vi "Create Status Queue.vi"(8 "error in (no error)":errorcluster, 11 "Test Step Controller.lvlib:Test Step Controller.lvclass":refnum<class "Server Controller.lvclass">) -> (0 "error out":errorcluster, 2 "queue out":refnum<queue>, 3 "Controller out":refnum<class "Server Controller.lvclass">)   [LabVIEW 2026, in "Server Controller.lvlib" / "Server Controller.lvclass"]
uses:
  Server Controller.lvclass
  Server Controller.lvclass/Server Controller.ctl
  MAL-Framework/user.lib/Common Components/Controller/Controller.lvclass
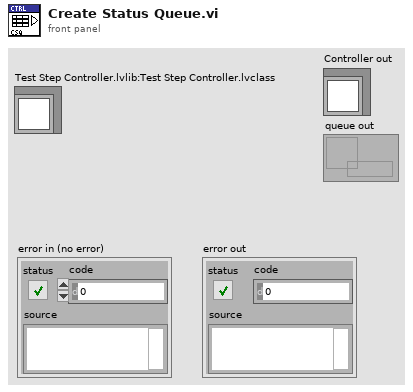
[diagram p1: front panel]
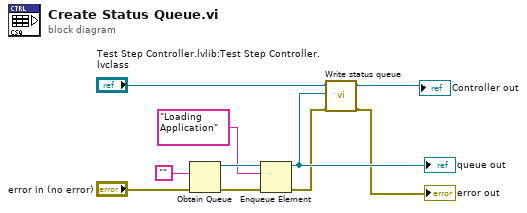
[diagram p0: block diagram]
diagram:
  n1 = Obtain Queue(element data type="", error in (no error)="error in (no error)") -> (queue out=w10:refnum<queue>, error out=w9:errorcluster)  [unwired: 3 in, 1 out]
  n2 = Enqueue Element(queue=w10, element="Loading Application" ("notification"), error in (no error)=w9) -> (queue out=w4:refnum<queue>, error out=w2:errorcluster)  [unwired: 1 in, 1 out]
  "queue out" <- w4
  n3 = call "Write status queue.vi"("error in (no error)"=w2, "status queue"=w4, "Controller in"="Test Step Controller.lvlib:Test Step Controller.lvclass") -> ("error out"=→"error out":errorcluster, "Controller out"=→"Controller out":refnum<class "Server Controller.lvclass">)  [unwired: 7 in]
